vi "1_05.vi"() -> ()   [LabVIEW 2018]
panel:
  in  "stop":bool
  out "Waveform Chart":dbl[](graph)
  in  "Amplitud":dbl=5.0
  in  "Frecuencia":dbl=1000.0
  in  "Muestras por segundo":dbl=2.0
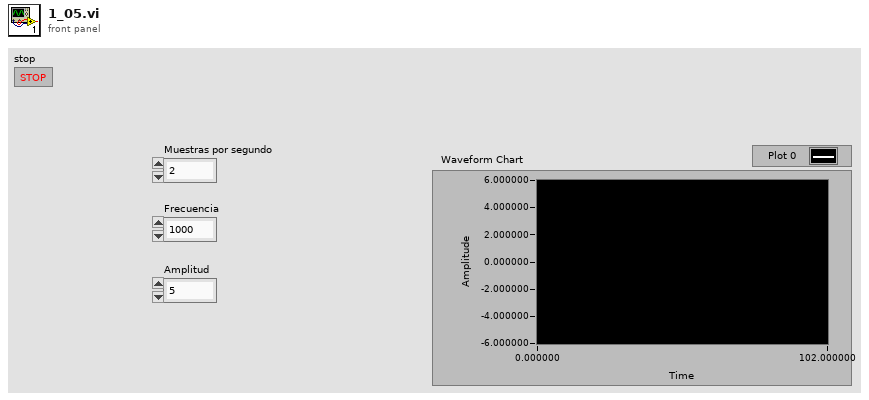
[diagram p1: front panel]
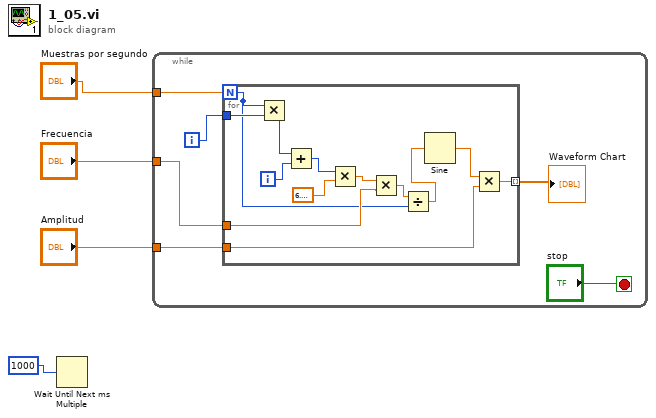
[diagram p0: block diagram]
diagram:
  n1 = Wait Until Next ms Multiple(millisecond multiple=1000) -> ()  [unwired: 1 out]
  n2 = while {
    tunnel: "Muestras por segundo" -> [w7]
    tunnel: "Amplitud" -> [w6]
    tunnel: "Frecuencia" -> [w5]
    i -> [w8]
    stop <- "stop" stop-if-true
    n3 = for {
      N: w7 -> [w12]
      tunnel: [w21] -> w10 mode=indexing
      tunnel: w8 -> [w20]
      tunnel: w6 -> [w16]
      tunnel: w5 -> [w14]
      i -> [w19]
      n4 = Multiply(x=w12, y=w20) -> (x*y=w18:i32)
      n5 = Add(x=w18, y=w19) -> (x+y=w17:i32)
      n6 = Multiply(x=w17, y=6.283185307179586) -> (x*y=w15:dbl)
      n7 = Multiply(x=w15, y=w14) -> (x*y=w13:dbl)
      n8 = Divide(x=w13, y=w12) -> (x/y=w11:dbl)
      n9 = Sine(x=w11) -> (sin(x)=w22:dbl)
      n10 = Multiply(x=w22, y=w16) -> (x*y=w21:dbl)
    }
    "Waveform Chart" <- w10
  }
